vi "clearpath_parse_differential_control.vi"(0 "ClearpathComm":T3) -> (1 "Data Valid?":bool=TRUE, 2 "Right Controls":T1, 3 "Left Controls":T2)   [LabVIEW 2012, in "clearpath_interface.lvlib"]
doc: "Parses differential control data (Message type 0x8201)"
uses:
  IGVC/Clearpath/Husky 2011/Teleop Robotics Project Folder/Husky/vi/clearpath_interface.lvlib
  cwrap_crio.dll
panel:
  # "Differential Controls"
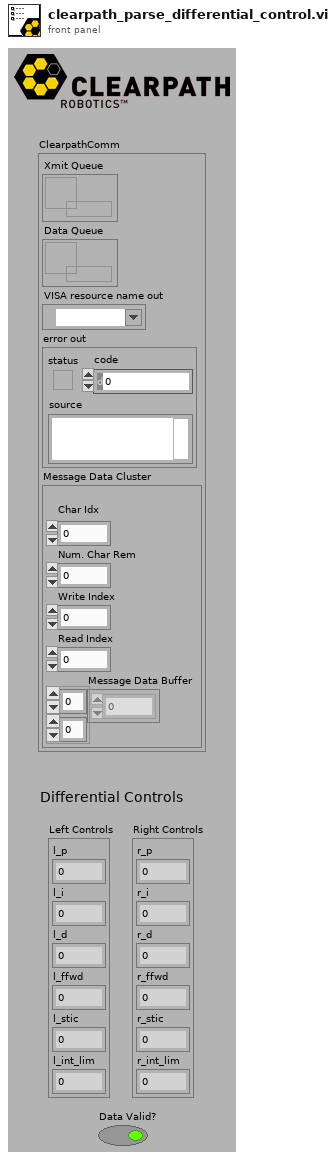
[diagram p1: front panel]
types:
  T1 = cluster{"r_p":dbl, "r_i":dbl, "r_d":dbl, "r_ffwd":dbl, "r_stic":dbl, "r_int_lim":dbl}
  T2 = cluster{"l_p":dbl, "l_i":dbl, "l_d":dbl, "l_ffwd":dbl, "l_stic":dbl, "l_int_lim":dbl}
  T3 = cluster{"Xmit Queue":refnum<queue>, "Data Queue":refnum<queue>, "VISA resource name out":refnum<visa-resource-name>, "error out":errorcluster, "Message Data Cluster":cluster{"\nChar Idx":u8, "Num. Char Rem":u8, "Write Index":u8, "Read Index":u8, "Message Data Buffer":u8[][]}}
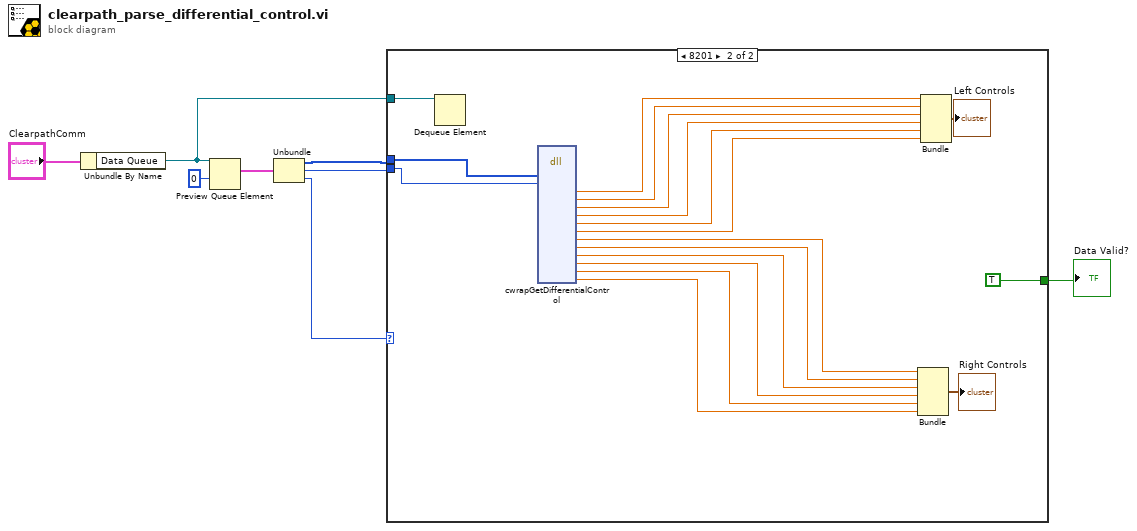
[diagram p0: block diagram]
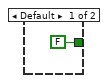
[diagram p2: hidden frame]
diagram:
  n1 = Unbundle By Name("ClearpathComm") -> ("Data Queue"=w1:refnum<queue>)
  n2 = Preview Queue Element(queue=w1, timeout in ms (-1)=0) -> (element=w6:cluster{u8[], "Length":i32, "Type":i32})  [unwired: 1 in, 3 out]
  n3 = Unbundle(w6) -> (w3:u8[], "Length"=w4:i32, "Type"=w5:i32)
  n4 = case shown="8201" w5 {
    tunnel: w4 -> [_ w26]
    tunnel: w3 -> [_ w27]
    tunnel: [FALSE TRUE] -> w2
    tunnel: w1 -> [_ w11]
    frame Default {
    }
    frame 33281 {
      n5 = Dequeue Element(queue=w11) -> ()  [unwired: 2 in, 4 out]
      n6 = dll-call lib="C:/Users/tebbeam/Documents/GitHub/IGVC-2013/Code/Project 1.0/Motors/Husky/cwrap_cRIO.*" fn="cwrapGetDifferentialControl"("packet"=w27, "len"=w26) -> ("l_p"=w14:dbl, "l_i"=w25:dbl, "l_d"=w24:dbl, "l_ffwd"=w23:dbl, "l_stic"=w22:dbl, "l_int_lim"=w21:dbl, "r_p"=w20:dbl, "r_i"=w19:dbl, "r_d"=w18:dbl, "r_ffwd"=w17:dbl, "r_stic"=w16:dbl, "r_int_lim"=w15:dbl)  [unwired: 18 in, 2 out]
      n7 = Bundle("r_p"=w20, "r_i"=w19, "r_d"=w18, "r_ffwd"=w17, "r_stic"=w16, "r_int_lim"=w15) -> (→"Right Controls":T1)  [unwired: 1 in]
      n8 = Bundle("l_p"=w14, "l_i"=w25, "l_d"=w24, "l_ffwd"=w23, "l_stic"=w22, "l_int_lim"=w21) -> (→"Left Controls":T2)  [unwired: 1 in]
    }
  }
  "Data Valid?" <- w2
